vi "Days Open Sort.vi"(11 "list in":T1[](array[typedef]) {"Creation Date" format="%<%x>T"; "Last Updated" format="%<%x>T"}) -> (3 "Array":T1[](array[typedef]) {"Creation Date" format="%<%x>T"; "Last Updated" format="%<%x>T"})   [LabVIEW 2018]
uses:
  Type Defs/SR Cluster.ctl
  Type Defs/SR Status.ctl
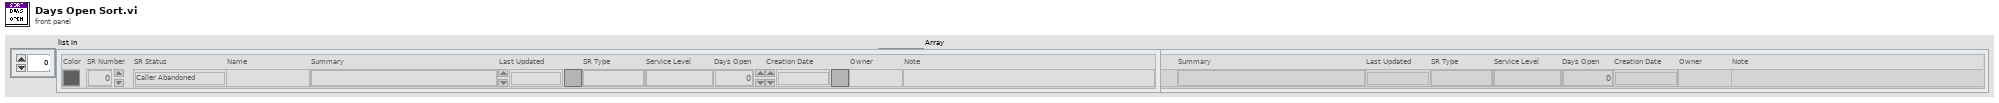
[diagram p1: front panel]
types:
  T1 = typedef "SR Cluster.ctl" = cluster{"Color":u32, "SR Number":i32, "SR Status":T2, "Name":string, "Summary":string, "Last Updated":timestamp, "SR Type":string, "Service Level":string, "Days Open":dbl, "Creation Date":timestamp, "Owner":string, "Note":string}
  T2 = typedef "SR Status.ctl" = enum16{"Caller Abandoned", "Created in Error", "Expired", "Forum Resolved AE", "Forum Resolved Customer", "IN WORK", "IN WORK Collab with AES", "IN WORK Collab with PSE", "IN WORK Collab with SE", "IN WORK Customer Added Note", "IN WORK Escalation", "IN WORK Wait on Customer", "Open", "Potentially Resolved", "Presumed Resolved", "RMA Approved for Return", "RMA Closed", "RMA Closed - DOA", "RMA In Progress", "RMA Open", "RMA Waiting on Customer", "Resolved", "Passed Off"}
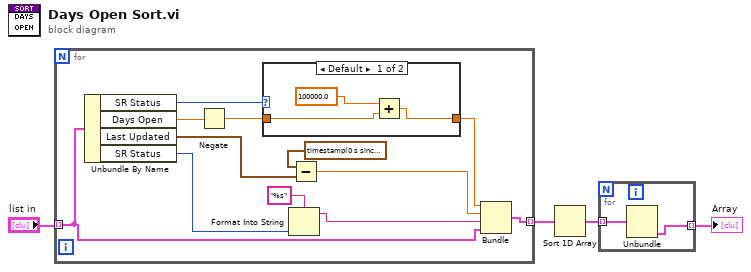
[diagram p0: block diagram]
diagram:
  n1 = for {
    tunnel: "list in" -> [w15] mode=indexing
    tunnel: [w16] -> w1 mode=indexing
    n2 = Unbundle By Name(w15) -> ("SR Status"=w8:T2, "Days Open"=w6:dbl, "Last Updated"=w13:timestamp, "SR Status"=w11:T2)
    n3 = Negate(x=w6) -> (-x=w5:dbl)
    n4 = case shown="Default" w8 {
      tunnel: [w18 w20] -> w7
      tunnel: w5 -> [w17 w20]
      frame Default {
        n5 = Add(x=100000.0, y=w17) -> (x+y=w18:dbl)
      }
      frame "IN WORK".."Open", "Passed Off" {
      }
    }
    n6 = Format Into String(format string="%s", w11) -> (resulting string=w9:string)  [unwired: 2 in, 1 out]
    n7 = Subtract(x=timestamp(0 s since 1904-01-01) ("Last Updated"), y=w13) -> (x-y=w12:dbl)
    n8 = Bundle(w7, w12, w9, "SR Cluster"=w15) -> (w16:cluster{dbl, dbl, string, "SR Cluster":T1})  [unwired: 1 in]
  }
  n9 = Sort 1D Array(array=w1) -> (sorted array=w2:cluster{dbl, dbl, string, "SR Cluster":T1}[])
  n10 = for {
    tunnel: w2 -> [w22] mode=indexing
    tunnel: [w21] -> w4 mode=indexing
    n11 = Unbundle(w22) -> ("SR Cluster"=w21:T1)  [unwired: 3 out]
  }
  "Array" <- w4
